vi "rewriteDataTDMS.vi"() -> ()   [LabVIEW 2019]
panel:
  in  "mix":path
  in  "karta":path
  in  "analizator":path
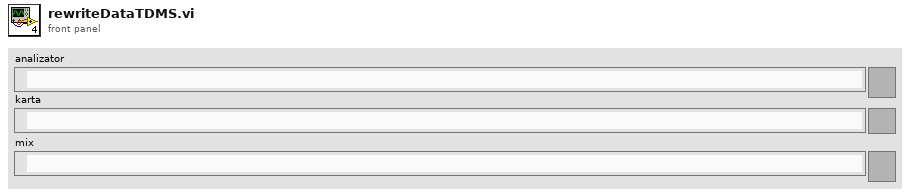
[diagram p1: front panel]
types:
  T1 = enum16{"open", "open or create", "create or replace", "create", "open (read-only)"}
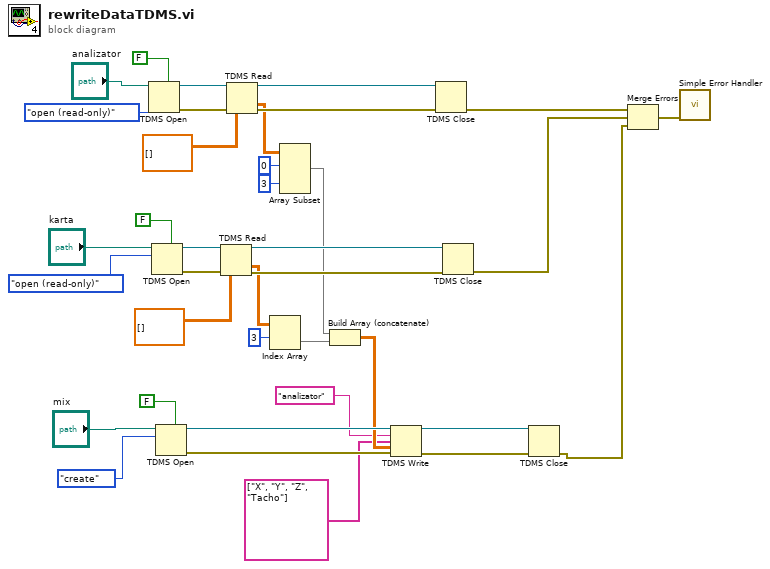
[diagram p0: block diagram]
diagram:
  n1 = TDMS Open(5:FALSE ("create index file? (T)"), 10:T1."open (read-only)" ("operation (0:open)"), 11:"analizator") -> (0:w33:errorcluster, 3:w34:refnum<k34>)  [unwired: 4 in]
  n2 = TDMS Open(5:FALSE ("create index file? (T)"), 10:T1."open (read-only)" ("operation (0:open)"), 11:"karta") -> (0:w29:errorcluster, 3:w30:refnum<k34>)  [unwired: 4 in]
  n3 = TDMS Open(5:FALSE ("create index file? (T)"), 10:T1."create" ("operation (0:open)"), 11:"mix") -> (0:w25:errorcluster, 3:w26:refnum<k34>)  [unwired: 4 in]
  n4 = TDMS Read(0:w30, 11:w29, 12:dbl[][] []) -> (4:w28:refnum<k34>, 10:w20:dbl[][], 15:w27:errorcluster)  [unwired: 5 in, 3 out]
  n5 = TDMS Read(0:w34, 11:w33, 12:dbl[][] []) -> (4:w32:refnum<k34>, 10:w18:dbl[][], 15:w31:errorcluster)  [unwired: 5 in, 3 out]
  n6 = Index Array(array=w20, index (row)=3) -> (element=w15:dbl[])  [unwired: 1 in]
  n7 = Array Subset(array=w18, index (row)=0 ("index"), length (row)=3 ("length")) -> (w14:dbl[][])  [unwired: 2 in]
  n8 = Build Array (concatenate)(w14, w15) -> (w13:dbl[][])
  n9 = TDMS Write(0:w26, 5:"analizator" ("group name in (Untitled)"), 7:string[] ["X", "Y", "Z", "Tacho"] ("channel name(s) in (Untitled)"), 9:w13, 11:w25) -> (4:w24:refnum<k34>, 15:w23:errorcluster)  [unwired: 1 in, 2 out]
  n10 = TDMS Close(8:w31, 11:w32) -> (0:w7:errorcluster)  [unwired: 1 out]
  n11 = TDMS Close(8:w27, 11:w28) -> (0:w5:errorcluster)  [unwired: 1 out]
  n12 = TDMS Close(8:w23, 11:w24) -> (0:w6:errorcluster)  [unwired: 1 out]
  n13 = Merge Errors(w7, w5, w6) -> (w4:errorcluster)
  n14 = call <vilib>:"Simple Error Handler.vi"("error in (no error)"=w4) -> ()  [unwired: 4 in, 5 out]
